vi "Untitled 9.vi"   [LabVIEW 2023]
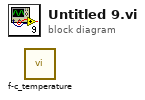
[diagram p0: block diagram]
diagram:
  n1 = call "f-c_temperature.vi"() -> ()  [unwired: 11 in, 1 out]
